vi "KillVi.vi"() -> ()   [LabVIEW 2016]
panel:
  in  "name or relative path":string="FrontPanel\\ZController.vi"
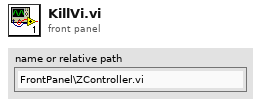
[diagram p1: front panel]
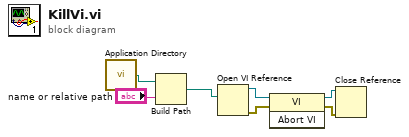
[diagram p0: block diagram]
diagram:
  n1 = call <vilib>:"Application Directory.vi"() -> ("Application Directory"=w6:path)
  n2 = Build Path(base path=w6, name or relative path="name or relative path") -> (appended path=w7:path)
  n3 = Open VI Reference(vi path=w7) -> (vi reference=w4:refnum<vi>, error out=w3:errorcluster)  [unwired: 5 in]
  n4 = invoke class="VI" method="Abort VI"(reference=w4, error in=w3) -> (reference out=w1:refnum<vi>, error out=w2:errorcluster)  [unwired: 1 in, 1 out]
  n5 = Close Reference(reference=w1, error in (no error)=w2) -> ()  [unwired: 1 out]
